vi "探头窗口-8-服务器版.vi"() -> ()   [LabVIEW 2013]
panel:
  in  "外部停止命令？":bool=TRUE
  out "引用-探头属性[]":refnum<vi>
  out "引用-监测模式？":refnum<vi>
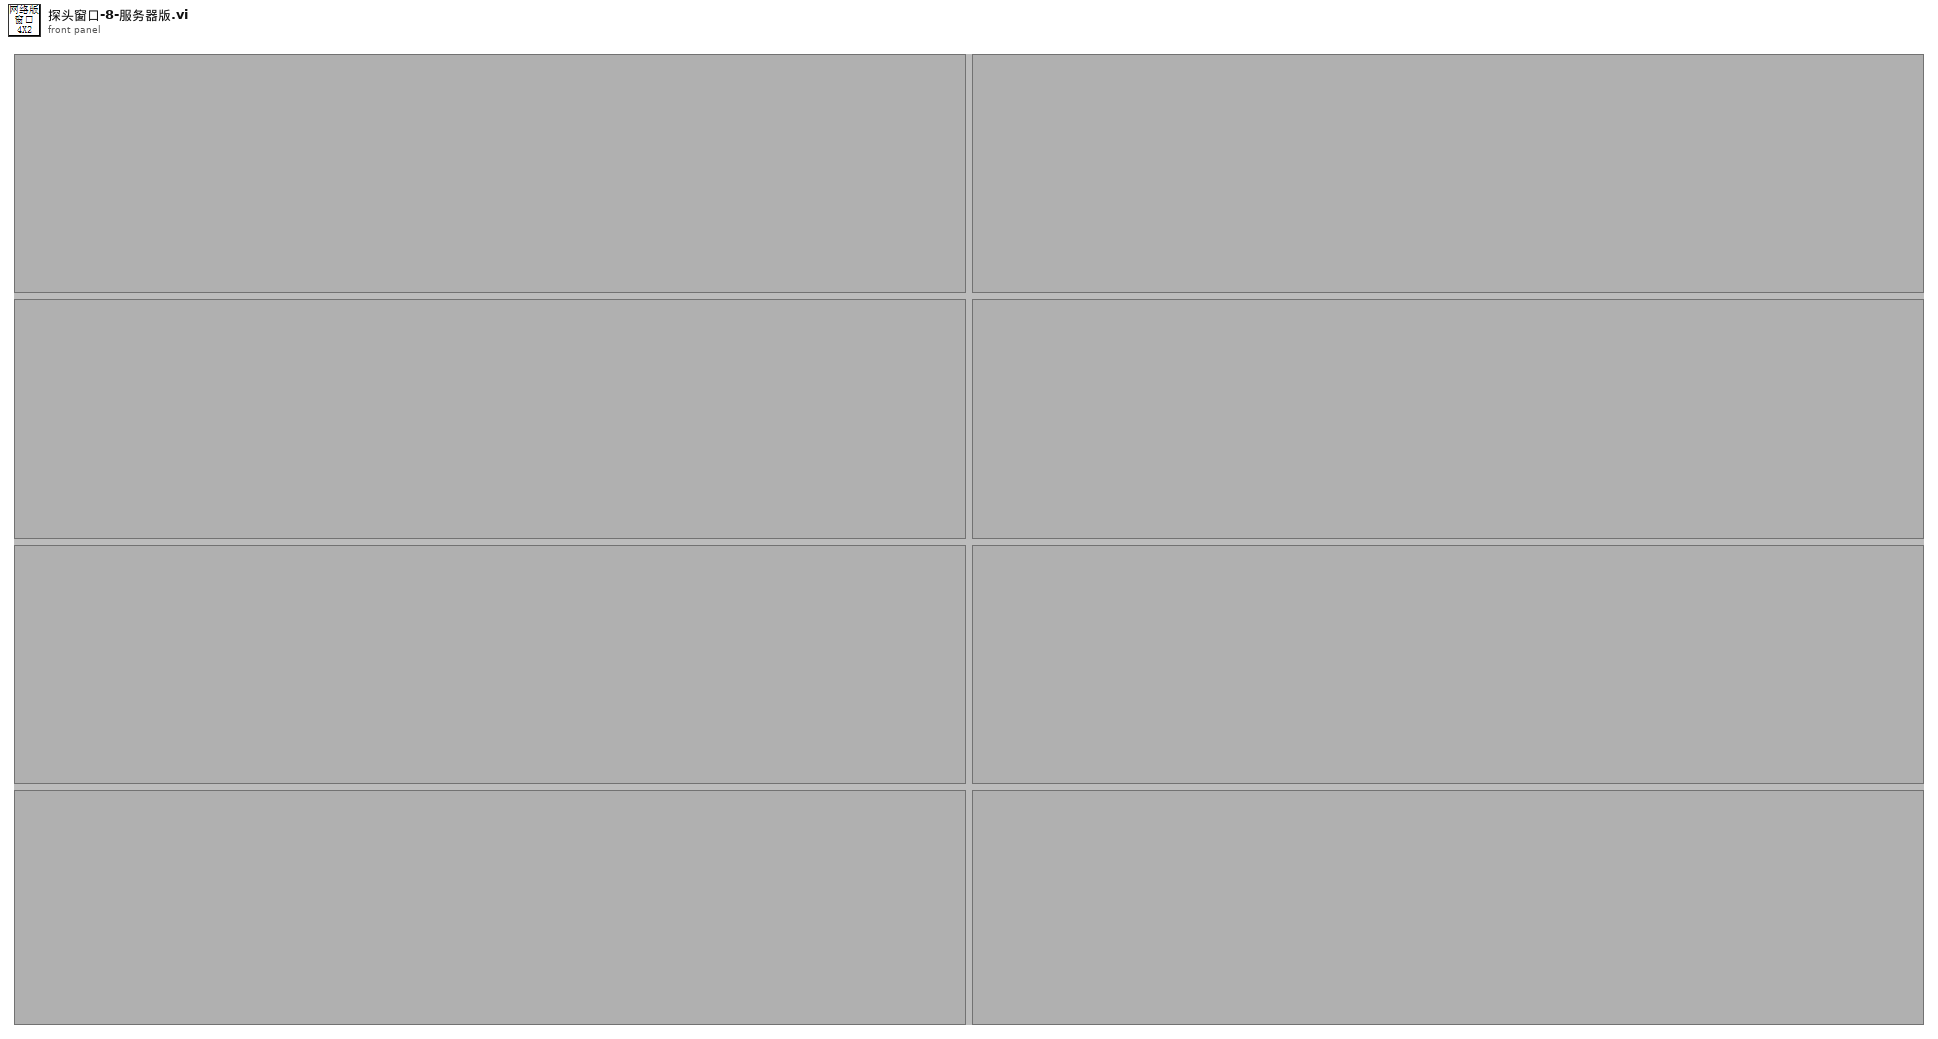
[diagram p1: front panel]
types:
  T1 = cluster{"探头地址与信息":cluster{"网络地址":cluster{"IP":string, "port":u16}, "探头信息":string}, "测量值":cluster{"时间":timestamp, "数值":dbl}, "限值":cluster{"限值1":dbl, "限值2":dbl}, "探头状态":enum16{"正常", "离线", "禁用", "一级报警", "二级报警"}}[]
  T2 = typedef "eventvkey.ctl" = enum16{"ASCII", "Enter", "Return", "Shift", "Ctrl", "Alt", "Cmd", "Opt", "Caps", "NumLock", "Clear", "Break", "Up", "Down", "Left", "Right", "Insert", "Delete", "Home", "End", "PageUp", "PageDown", "Escape", "Help", "Pause", "ScrollLock", "F1", "F2", "F3", "F4", "F5", "F6", "F7", "F8", "F9", "F10", "F11", "F12", "F13", "F14", "F15", "F16", "F17", "F18", "F19", "F20", "F21", "F22", "F23", "F24", "Play", "VolumeUp", "VolumeDown", "Mute", "Two Byte Char"}
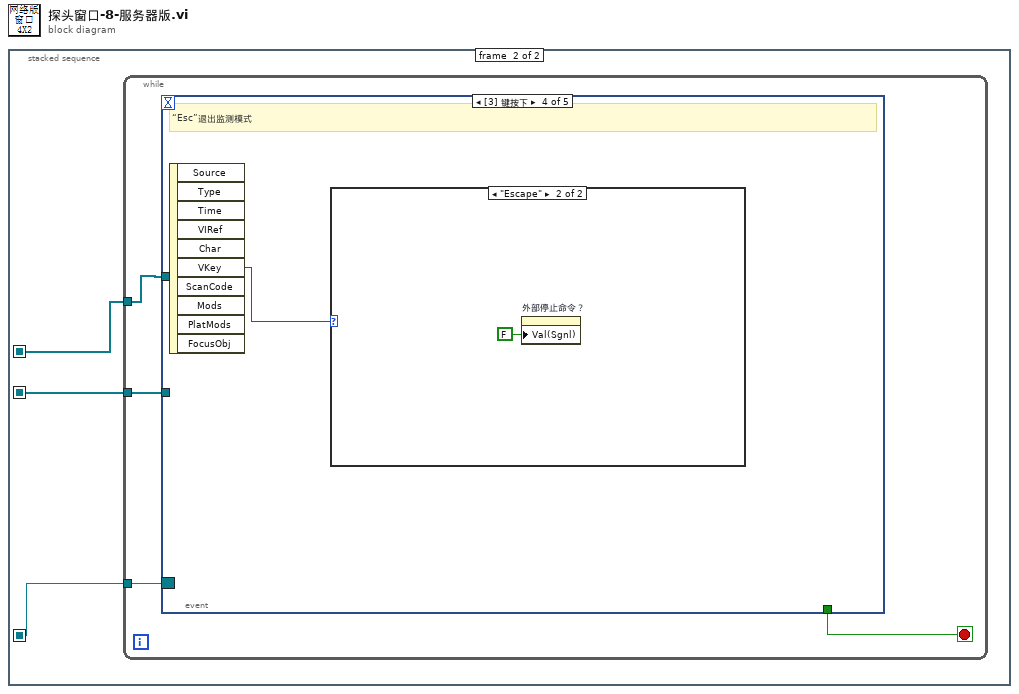
[diagram p0: block diagram]
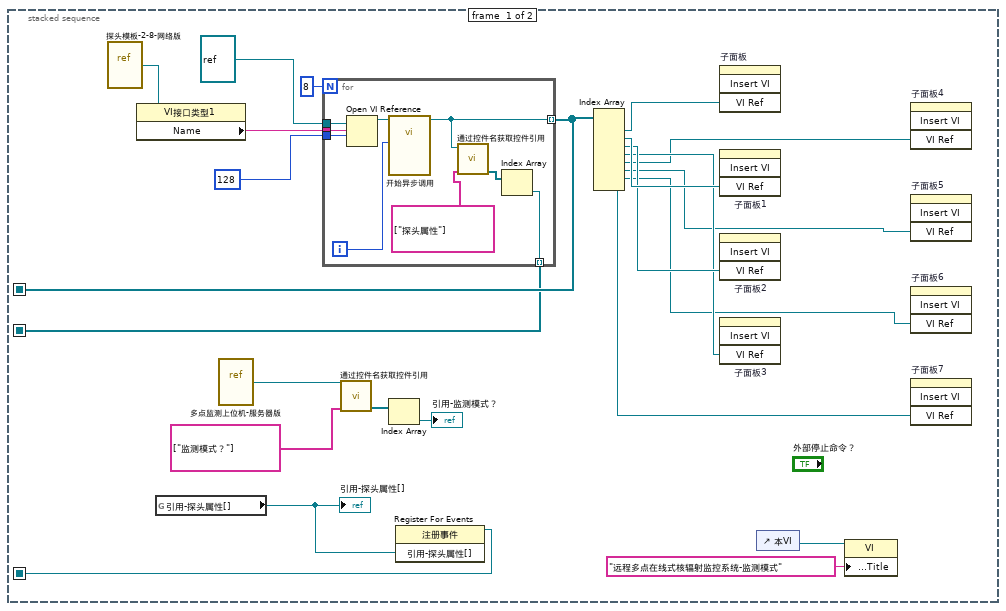
[diagram p2: hidden frame]
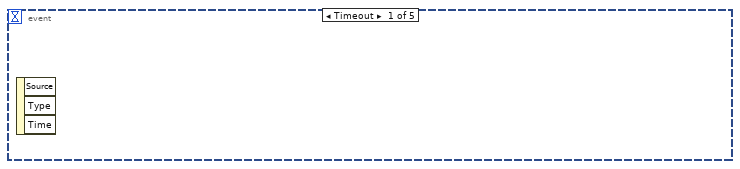
[diagram p3: hidden frame]
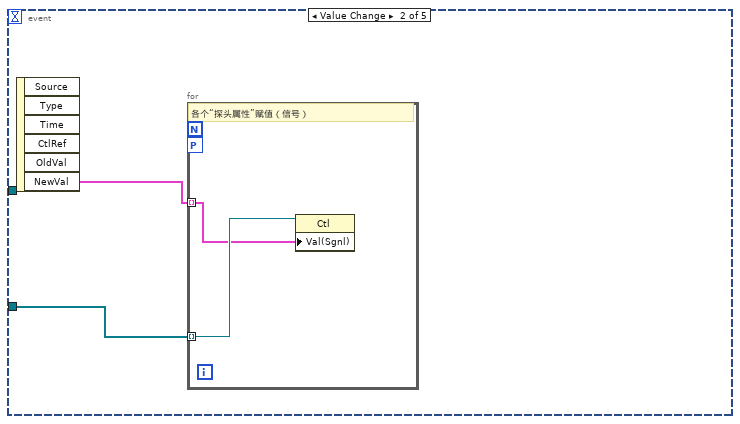
[diagram p4: hidden frame]
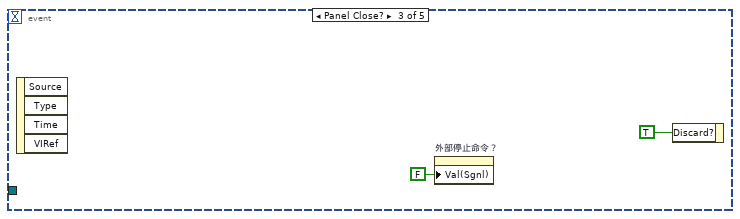
[diagram p5: hidden frame]
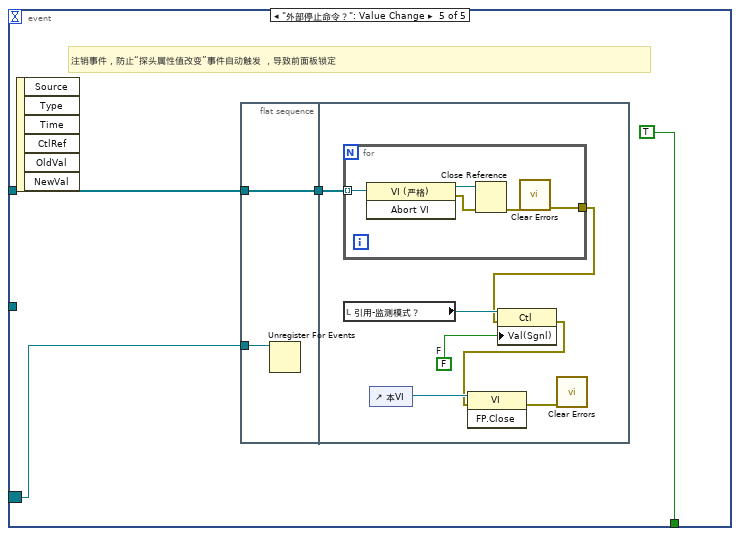
[diagram p7: hidden frame]
diagram:
  n1 = stacked-sequence {
    seq-local: [w19 _] -> [_ w35]
    seq-local: [w17 _] -> [_ w34]
    seq-local: [w3 _] -> [_ w33]
    frame #0 {
      n2 = vi-ref "探头模板-2-8-网络版.vi"() -> (w23:refnum<vi>)
      n3 = property class="VI接口类型1"(reference=w23) -> ("Name"=w22:string)  [unwired: 1 in, 2 out]
      n4 = global read "全局变量-35点监测.vi" "引用-探头属性[]"() -> (w4:refnum<vi>)
      "引用-探头属性[]" <- w4
      n5 = vi-ref "多点监测上位机-服务器版.vi"() -> (w5:refnum<vi>)
      n6 = for {
        N: 8 -> [_]
        tunnel: w22 -> [w32]
        tunnel: 128 ("选项") -> [w31]
        tunnel: refnum<vi> refnum ("类型说明符VI引用句柄（仅用于类型）") -> [w30]
        tunnel: [w25] -> w19 mode=indexing
        tunnel: [w26] -> w17 mode=indexing
        i -> [w24]
        n7 = Open VI Reference(type specifier VI Refnum (for type only)=w30, vi path=w32, options=w31) -> (vi reference=w27:refnum<vi>)  [unwired: 3 in, 1 out]
        n8 = call-by-ref "开始异步调用"(reference=w27, "探头序号"=w24) -> (reference out=w25:refnum<vi>)  [unwired: 12 in, 1 out]
        n9 = call "通过控件名获取控件引用.vi"("控件名数组"=string[] ["探头属性"], "VI引用"=w25) -> ("控件引用输出"=w29:refnum<vi>[])  [unwired: 7 in, 2 out]
        n10 = Index Array(array=w29) -> (element=w26:refnum<vi>)  [unwired: 1 in]
      }
      n11 = call "通过控件名获取控件引用.vi"("控件名数组"=string[] ["监测模式？"], "VI引用"=w5) -> ("控件引用输出"=w7:refnum<vi>[])  [unwired: 7 in, 2 out]
      n12 = Index Array(array=w7) -> (element=→"引用-监测模式？":refnum<vi>)  [unwired: 1 in]
      n13 = register-events(w4) -> (reference out=w3:refnum<event-registration>)  [unwired: 2 in, 1 out]
      n14 = Index Array(array=w19) -> (element #1=w16:refnum<vi>, element #2=w15:refnum<vi>, element #3=w14:refnum<vi>, element #4=w13:refnum<vi>, element #5=w12:refnum<vi>, element #6=w11:refnum<vi>, element #7=w10:refnum<vi>, element #8=w9:refnum<vi>)  [unwired: 8 in]
      n15 = invoke on="子面板" class="SubPnl" method="Insert VI"("VI Ref"=w16) -> ()  [unwired: 3 in, 4 out]
      n16 = invoke on="子面板1" class="SubPnl" method="Insert VI"("VI Ref"=w15) -> ()  [unwired: 3 in, 4 out]
      n17 = invoke on="子面板2" class="SubPnl" method="Insert VI"("VI Ref"=w14) -> ()  [unwired: 3 in, 4 out]
      n18 = invoke on="子面板3" class="SubPnl" method="Insert VI"("VI Ref"=w13) -> ()  [unwired: 3 in, 4 out]
      n19 = control-ref of="本VI"() -> (w2:refnum<vi>)
      n20 = property class="VI"(reference=w2, "Front Panel.Title"="远程多点在线式核辐射监控系统-监测模式" ("前面板窗口:标题")) -> ()  [unwired: 1 in, 2 out]
      n21 = invoke on="子面板4" class="SubPnl" method="Insert VI"("VI Ref"=w12) -> ()  [unwired: 3 in, 4 out]
      n22 = invoke on="子面板5" class="SubPnl" method="Insert VI"("VI Ref"=w11) -> ()  [unwired: 3 in, 4 out]
      n23 = invoke on="子面板6" class="SubPnl" method="Insert VI"("VI Ref"=w10) -> ()  [unwired: 3 in, 4 out]
      n24 = invoke on="子面板7" class="SubPnl" method="Insert VI"("VI Ref"=w9) -> ()  [unwired: 3 in, 4 out]
    }
    frame #1 {
      n25 = while {
        tunnel: w35 -> [w38]
        tunnel: w34 -> [w37]
        tunnel: w33 -> [w36]
        stop <- w39 stop-if-true
        n26 = event shown="[3] 键按下" {
          selector: w36 -> [_ _ _ _ w48]
          dyn-events: _ -> [_ _ _ _ _]
          timeout: _ -> [_ _ _ _ _]
          tunnel: [_ _ _ _ TRUE ("放弃？")] -> w39
          tunnel: w38 -> [_ _ _ _ w50]
          tunnel: w37 -> [_ w40 _ _ _]
          event Timeout {
            n27 = event-data() -> ()  [unwired: 1 in, 3 out]
          }
          event Value Change {
            n28 = event-data() -> ("NewVal"=w41:T1)  [unwired: 1 in, 5 out]
            n29 = for {
              workers-P: _ -> [_]
              tunnel: w40 -> [w43] mode=indexing
              tunnel: w41 -> [w42] mode=indexing
              # "各个“探头属性”赋值（信号）"
              n30 = property class="Ctl"(reference=w43, "Val(Sgnl)"=w42) -> ()  [unwired: 1 in, 2 out]
            }
          }
          event Panel Close? {
            n31 = event-data() -> ()  [unwired: 1 in, 4 out]
            n32 = property on="外部停止命令？" class="Bool (严格)"("Val(Sgnl)"=FALSE ("值(信号)")) -> ()  [unwired: 2 in, 2 out]
            n33 = event-data("Discard?"=TRUE ("放弃？")) -> ()  [unwired: 1 in, 1 out]
          }
          event Key Down {
            # "“Esc”退出监测模式"
            n34 = event-data() -> ("VKey"=w46:T2)  [unwired: 1 in, 9 out]
            n35 = case shown="\"Escape\"" w46 {
              frame "ASCII", Default {
              }
              frame "Escape" {
                n36 = property on="外部停止命令？" class="Bool (严格)"("Val(Sgnl)"=FALSE ("值(信号)")) -> ()  [unwired: 2 in, 2 out]
              }
            }
          }
          event "外部停止命令？": Value Change {
            # "注销事件，防止“探头属性值改变”事件自动触发 ，导致前面板锁定"
            n37 = event-data() -> ()  [unwired: 1 in, 6 out]
            n38 = flat-sequence {
              tunnel: w50 -> [w53]
              tunnel: [w53] -> w49
              tunnel: w48 -> [w52]
              tunnel: w49 -> [w60]
              frame #0 {
                n39 = Unregister For Events(event registration refnum=w52) -> ()  [unwired: 1 in, 1 out]
              }
              frame #1 {
                w59 = FALSE  # F
                n40 = for {
                  tunnel: w60 -> [w65] mode=indexing
                  tunnel: [w61] -> w56
                  n41 = invoke class="VI (严格)" method="Abort VI"(reference=w65) -> (reference out=w63:refnum<vi>, error out=w64:errorcluster)  [unwired: 2 in, 1 out]
                  n42 = Close Reference(reference=w63, error in (no error)=w64) -> (error out=w62:errorcluster)
                  n43 = call <vilib>:"Clear Errors.vi"("error in (no error)"=w62) -> ("error out"=w61:errorcluster)  [unwired: 6 in]
                }
                n44 = local read "引用-监测模式？"() -> (w58:refnum<vi>)
                n45 = control-ref of="本VI"() -> (w57:refnum<vi>)
                n46 = property class="Ctl"(reference=w58, error in=w56, "Val(Sgnl)"=w59) -> (error out=w55:errorcluster)  [unwired: 1 out]
                n47 = invoke class="VI" method="FP.Close"(reference=w57, error in=w55) -> (error out=w54:errorcluster)  [unwired: 1 in, 2 out]
                n48 = call <vilib>:"Clear Errors.vi"("error in (no error)"=w54) -> ()  [unwired: 6 in, 1 out]
              }
            }
          }
        }
      }
    }
  }
